vi "Set Connection Status.vi"(8 "error in (no error)":errorcluster, 11 "connected":bool) -> (0 "error out":errorcluster)   [LabVIEW 2021, in "AudioGenManageConnectionProcess.lvlib"]
uses:
  AudioGenManageConnectionProcess.lvlib
  <vilib>/addons/PointValueMap/subVIs/Point_Write_variant.vi
  <vilib>/addons/PointValueMap/PointValueMap.lvlib
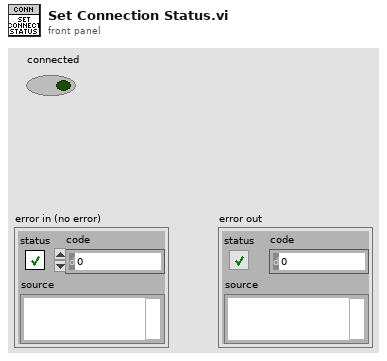
[diagram p1: front panel]
types:
  T1 = typedef "PointValueMap.lvlib/PointMap.ctl" = refnum<data-value>
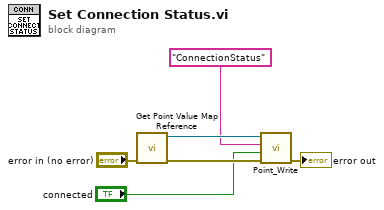
[diagram p0: block diagram]
diagram:
  n1 = call "Get Point Value Map Reference.vi"("error in (no error)"="error in (no error)") -> ("error out"=w4:errorcluster, "Map Out"=w5:T1)  [unwired: 9 in]
  n2 = call-poly <vilib>:"Point_Write.vi"("Error In"=w4, "Value"="connected", "Tag"="ConnectionStatus", "Map"=w5) -> ("Error Out"=→"error out":errorcluster)  [unwired: 6 in, 1 out]
